vi "CF-store_error.vi"(7 "Location":string, 8 "error in (no error)":errorcluster) -> ()   [LabVIEW 2020, in "CF-common_features.lvlib"]
uses:
  CF-common_features.lvlib
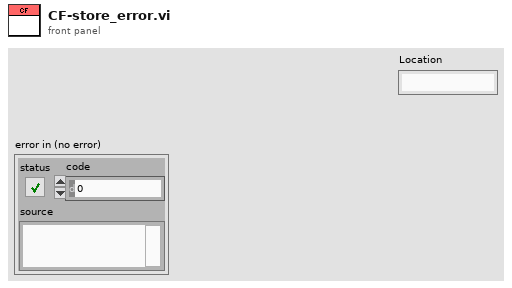
[diagram p1: front panel]
types:
  T1 = enum16{"open", "replace", "create", "open or create", "replace or create", "replace or create with confirmation"}
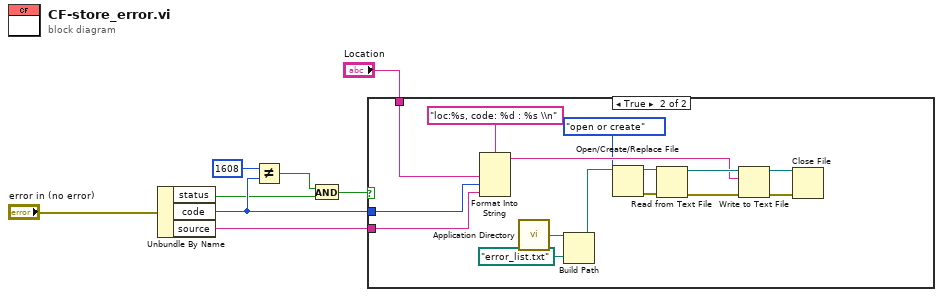
[diagram p0: block diagram]
diagram:
  n1 = Unbundle By Name("error in (no error)") -> ("status"=w3:bool, "code"=w5:i32, "source"=w7:string)
  n2 = Not Equal?(x=1608, y=w5) -> (x != y?=w2:bool)
  n3 = And(x=w2, y=w3) -> (x .and. y?=w1:bool)
  n4 = case shown="True" w1 {
    tunnel: w5 -> [_ w10]
    tunnel: w7 -> [_ w9]
    tunnel: "Location" -> [_ w14]
    frame False {
    }
    frame True {
      n5 = Format Into String(format string="loc:%s, code: %d : %s \\n", w14, w10, w9) -> (resulting string=w13:string)  [unwired: 2 in, 1 out]
      n6 = call <vilib>:"Application Directory.vi"() -> ("Application Directory"=w16:path)
      n7 = Build Path(base path=w16, name or relative path=path "error_list.txt") -> (appended path=w15:path)
      n8 = Open/Create/Replace File(file path (use dialog)=w15, operation (0:open)=T1."open or create") -> (refnum out=w22:refnum<file>, error out=w21:errorcluster)  [unwired: 4 in, 1 out]
      n9 = Read from Text File(file (use dialog)=w22, error in=w21) -> (refnum out=w20:refnum<file>, error out=w19:errorcluster)  [unwired: 2 in, 2 out]
      n10 = Write to Text File(file (use dialog)=w20, text=w13, error in=w19) -> (refnum out=w18:refnum<file>, error out=w17:errorcluster)  [unwired: 1 in, 1 out]
      n11 = Close File(refnum=w18, error in=w17) -> ()  [unwired: 2 out]
    }
  }
